vi "Peak Detector (multiple).vi"(6 "Width Units (points)":enum16{"Points", "Data"}(ring), 8 "error in (no error)":errorcluster, 9 "width":dbl=3.0 min=3.0, 10 "threshold":dbl format="%0.2f", 11 "XY-data":cluster{"X-array":dbl[], "Y-array":dbl[]}[](array[cluster])) -> (0 "error out":errorcluster, 1 "Amplitudes":cluster{"Amplitudes":dbl[]}[](array[cluster]), 2 "Locations":cluster{"Locations":dbl[]}[](array[cluster]), 3 "XY-data out":cluster{"X-array":dbl[], "Y-array":dbl[]}[](array[cluster]) {"Y-array" format="%.2p"; "X-array" format="%.2p"})   [LabVIEW 2016, in "xy_utilities.lvlib"]
doc: "Find <b>peaks</b> in <b>XY-data</b>'s Y-Array.\n\nWire data to the data input to determine the polymorphic instance to use or manually select the instance."
uses:
  xy_utilities.lvlib
  Private/h.vi
  Private/X Array Range to Index.vi
  <vilib>/Utility/error.llb/Error Cluster From Error Code.vi
  <userlib>/_MGI/1D Array/MGI Interpolate 1D Array Extended.vi
  <vilib>/Analysis/8numeric.llb/Peak Detector.vi
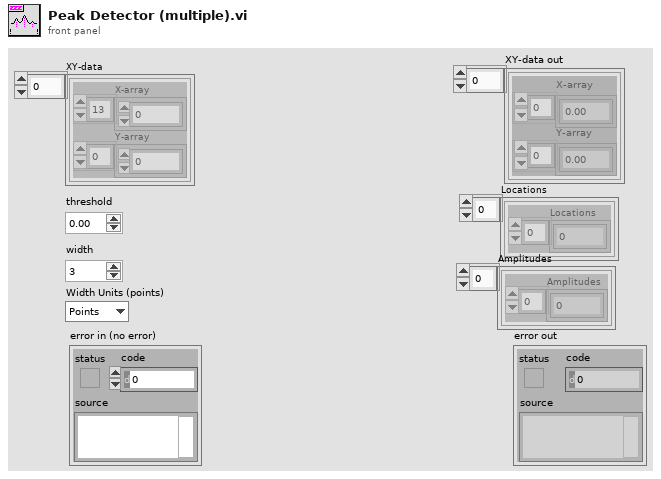
[diagram p1: front panel]
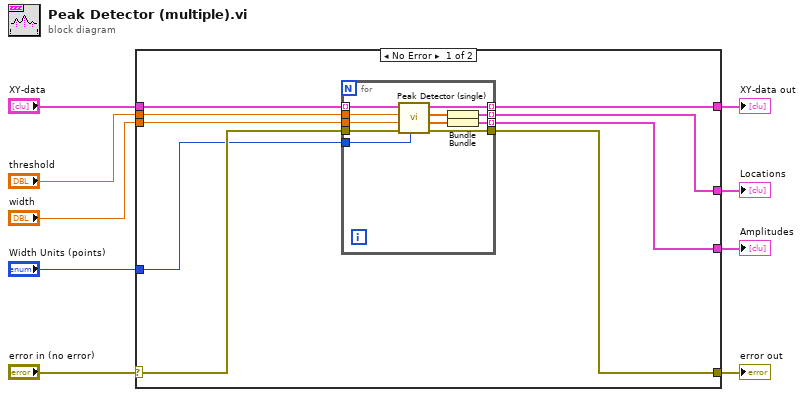
[diagram p0: block diagram]
diagram:
  n1 = case shown="No Error" "error in (no error)" {
    selector: "error in (no error)" -> [w16 w31]
    tunnel: [w15 w31] -> w8
    tunnel: "XY-data" -> [w18 w30]
    tunnel: [w17 w30] -> w6
    tunnel: "width" -> [w14 _]
    tunnel: "threshold" -> [w13 _]
    tunnel: [w12 _] -> w3
    tunnel: [w11 _] -> w2
    tunnel: "Width Units (points)" -> [w10 _]
    frame No Error {
      n2 = for {
        tunnel: w18 -> [w29] mode=indexing
        tunnel: [w27] -> w17 mode=indexing
        tunnel: w16 -> [w28]
        tunnel: [w26] -> w15
        tunnel: w14 -> [w25]
        tunnel: w13 -> [w24]
        tunnel: [w21] -> w12 mode=indexing
        tunnel: [w20] -> w11 mode=indexing
        tunnel: w10 -> [w19]
        n3 = call "Peak Detector (single).vi"("Width Units (points)"=w19, "error in (no error)"=w28, "width"=w25, "threshold"=w24, "XY-data"=w29) -> ("error out"=w26:errorcluster, "Amplitudes"=w22:dbl[], "Locations"=w23:dbl[], "XY-data out"=w27:cluster{"X-array":dbl[], "Y-array":dbl[]})  [unwired: 3 in]
        n4 = Bundle("Locations"=w23) -> (w21:cluster{"Locations":dbl[]})  [unwired: 1 in]
        n5 = Bundle("Amplitudes"=w22) -> (w20:cluster{"Amplitudes":dbl[]})  [unwired: 1 in]
      }
    }
    frame Error {
    }
  }
  "error out" <- w8
  "XY-data out" <- w6
  "Locations" <- w3
  "Amplitudes" <- w2
